vi "Read id.vi"(8 "error in (no error)":errorcluster, 11 "TestInterface in":refnum<class "TestInterface.lvclass">) -> (0 "error out":errorcluster, 2 "id":u32, 3 "TestInterface out":refnum<class "TestInterface.lvclass">)   [LabVIEW 2013, in "TestInterface.lvclass"]
uses:
  TestInterface.lvclass
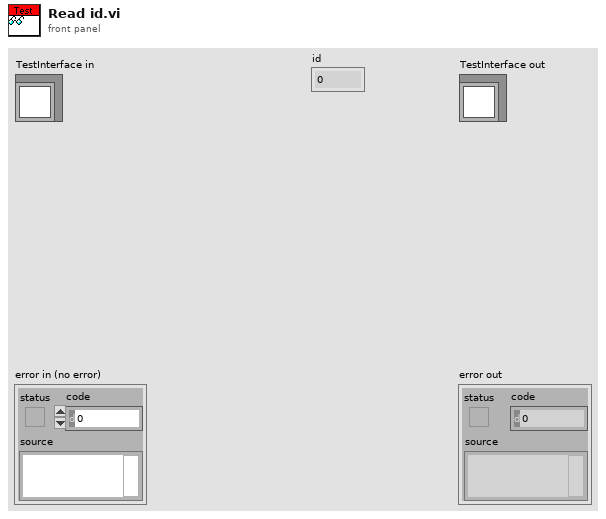
[diagram p1: front panel]
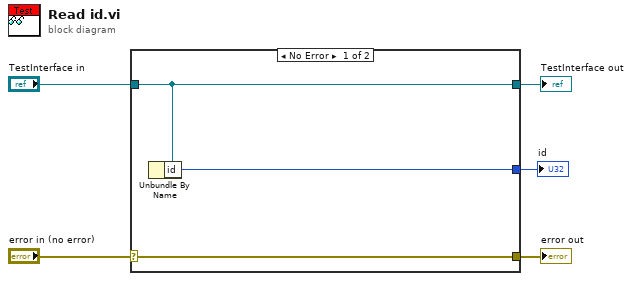
[diagram p0: block diagram]
diagram:
  n1 = case shown="No Error" "error in (no error)" {
    selector: "error in (no error)" -> [w8 w9]
    tunnel: [w8 w9] -> w4
    tunnel: [w7 w10] -> w2
    tunnel: "TestInterface in" -> [w7 w10]
    tunnel: [w6 _] -> w1
    frame No Error {
      n2 = Unbundle By Name(w7) -> ("id"=w6:u32)
    }
    frame Error {
    }
  }
  "error out" <- w4
  "TestInterface out" <- w2
  "id" <- w1
